vi "Create New VI from Template.vi"   [LabVIEW 2017]
doc: "Creates new VI from BenjaminR's VI Template."
types:
  T1 = enum32{"Invalid", "Standard", "Closed", "Hidden", "Minimized", "Maximized"}
  T2 = enum32{"invalid VI type", "Standard VI", "Control VI", "Global VI", "Polymorphic VI", "Configuration VI", "SubSystem", "Facade VI", "Method VI", "Statechart Diagram VI"}
  T3 = typedef "LVRectTypeDef.ctl" = cluster{"Left":i16, "Top":i16, "Right":i16, "Bottom":i16}
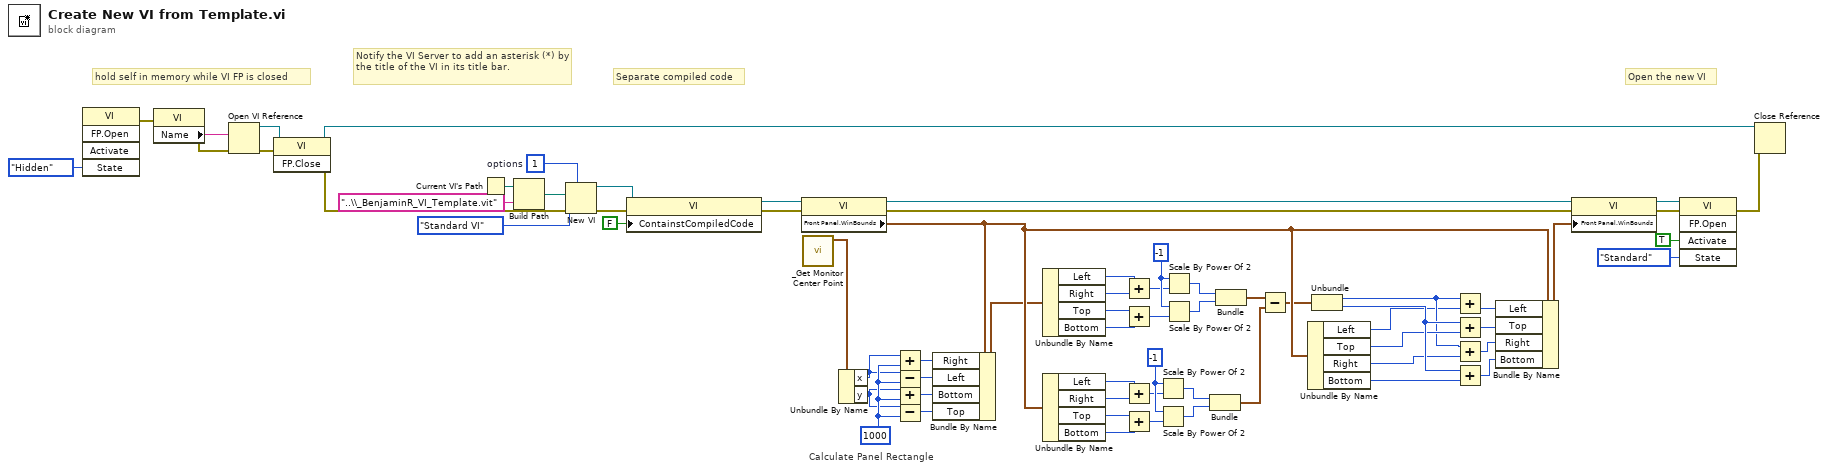
[diagram p0: block diagram]
diagram:
  w17 = -1
  w26 = -1
  w34 = 1000 ("x")
  w52 = u32 1  # options
  # "Calculate Panel Rectangle"
  # "Open the new VI"
  # "Separate compiled code"
  # "Notify the VI Server to add an asterisk (*) by the title of the VI in its title bar."
  # "hold self in memory while VI FP is closed"
  n1 = invoke class="VI" method="FP.Open"("State"=T1."Hidden") -> (error out=w59:errorcluster)  [unwired: 4 in, 4 out]
  n2 = property class="VI"(error in=w59) -> (error out=w60:errorcluster, "Name"=w64:string)  [unwired: 1 in, 1 out]
  n3 = Open VI Reference(vi path=w64, error in (no error)=w60) -> (vi reference=w63:refnum<vi>, error out=w62:errorcluster)  [unwired: 4 in]
  n4 = invoke class="VI" method="FP.Close"(reference=w63, error in=w62) -> (reference out=w57:refnum<vi>, error out=w58:errorcluster)  [unwired: 1 in, 1 out]
  n5 = Current VI's Path() -> (path=w67:path)
  n6 = Build Path(base path=w67, name or relative path="..\\_BenjaminR_VI_Template.vit") -> (appended path=w65:path)
  n7 = New VI(7:w52, 8:w58, 9:T2."Standard VI" ("vi type (standard vi)"), 10:w65) -> (0:w55:errorcluster, 3:w54:refnum<vi>)  [unwired: 3 in]
  n8 = property class="VI"(reference=w54, error in=w55, "ContainstCompiledCode"=FALSE ("Contains Compiled Code")) -> (reference out=w42:refnum<vi>, error out=w43:errorcluster)
  n9 = property class="VI"(reference=w42, error in=w43) -> (reference out=w48:refnum<vi>, error out=w44:errorcluster, "Front Panel.WinBounds"=w46:T3)
  n10 = call "_Get Monitor Center Point.vi"() -> ("Center"=w47:cluster{"x":i32, "y":i32})  [unwired: 11 in]
  n11 = Unbundle By Name(w47) -> ("x"=w32:i32, "y"=w33:i32)
  n12 = Add(x=w32, y=w34) -> (x+y=w36:i32)
  n13 = Subtract(x=w32, y=w34) -> (x-y=w37:i32)
  n14 = Add(x=w33, y=w34) -> (x+y=w38:i32)
  n15 = Subtract(x=w33, y=w34) -> (x-y=w39:i32)
  n16 = Bundle By Name(cluster=w46, "Right"=w36, "Left"=w37, "Bottom"=w38, "Top"=w39) -> (w35:T3)
  n17 = Unbundle By Name(w35) -> ("Left"=w11:i16, "Right"=w12:i16, "Top"=w13:i16, "Bottom"=w14:i16)
  n18 = Unbundle By Name(w46) -> ("Left"=w20:i16, "Right"=w21:i16, "Top"=w22:i16, "Bottom"=w23:i16)
  n19 = Add(x=w11, y=w12) -> (x+y=w16:i16)
  n20 = Add(x=w13, y=w14) -> (x+y=w15:i16)
  n21 = Add(x=w20, y=w21) -> (x+y=w25:i16)
  n22 = Add(x=w22, y=w23) -> (x+y=w24:i16)
  n23 = Scale By Power Of 2(n=w26, x=w25) -> (x*2^n=w27:i16)
  n24 = Scale By Power Of 2(n=w26, x=w24) -> (x*2^n=w28:i16)
  n25 = Scale By Power Of 2(n=w17, x=w16) -> (x*2^n=w18:i16)
  n26 = Scale By Power Of 2(n=w17, x=w15) -> (x*2^n=w19:i16)
  n27 = Bundle(w27, w28) -> (w30:cluster{i16, i16})  [unwired: 1 in]
  n28 = Bundle(w18, w19) -> (w29:cluster{i16, i16})  [unwired: 1 in]
  n29 = Subtract(x=w29, y=w30) -> (x-y=w31:cluster{i16, i16})
  n30 = Unbundle By Name(w46) -> ("Left"=w1:i16, "Top"=w6:i16, "Right"=w3:i16, "Bottom"=w8:i16)
  n31 = Unbundle(w31) -> (w4:i16, w7:i16)
  n32 = Add(x=w4, y=w1) -> (x+y=w2:i16)
  n33 = Add(x=w7, y=w6) -> (x+y=w10:i16)
  n34 = Add(x=w4, y=w3) -> (x+y=w5:i16)
  n35 = Add(x=w7, y=w8) -> (x+y=w9:i16)
  n36 = Bundle By Name(cluster=w46, "Left"=w2, "Top"=w10, "Right"=w5, "Bottom"=w9) -> (w45:T3)
  n37 = property class="VI"(reference=w48, error in=w44, "Front Panel.WinBounds"=w45) -> (reference out=w41:refnum<vi>, error out=w40:errorcluster)
  n38 = invoke class="VI" method="FP.Open"(reference=w41, error in=w40, "Activate"=TRUE ("Activate?"), "State"=T1."Standard") -> (error out=w51:errorcluster)  [unwired: 1 in, 4 out]
  n39 = Close Reference(reference=w57, error in (no error)=w51) -> ()  [unwired: 1 out]
